vi "Insert LogData in Q.vi"(8 "error in (no error)":errorcluster, 10 "EventLog":T1) -> (0 "error out":errorcluster, 2 "# elements in queue":i32, 3 "EventLogDataQRef":refnum<queue>)   [LabVIEW 2022 SP3]
doc: "Developed by Kevin Thompson\nThompson Engineering, LLC\nkevin@thompsonengineering.net"
uses:
  TD EventLogData--cluster.ctl
  GBL DataQ Ref.vi
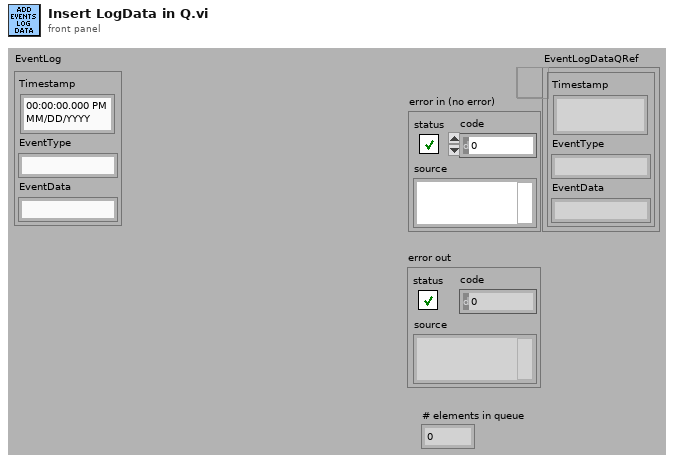
[diagram p1: front panel]
types:
  T1 = typedef "TD EventLogData--cluster.ctl" = cluster{"Timestamp":timestamp, "EventType":string, "EventData":string}
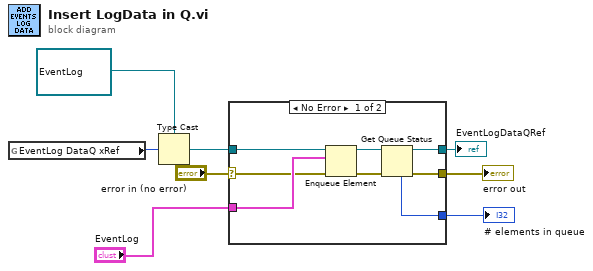
[diagram p0: block diagram]
diagram:
  n1 = global read "GBL DataQ Ref.vi" "EventLog DataQ xRef"() -> (w5:u32)
  n2 = Type Cast(type=refnum<queue> refnum ("EventLogDataQRef"), x=w5) -> (*(type *) &x=w6:refnum<queue>)
  n3 = case shown="No Error" "error in (no error)" {
    selector: "error in (no error)" -> [w13 w17]
    tunnel: w6 -> [w15 w18]
    tunnel: [w10 w17] -> w8
    tunnel: [w12 w18] -> w1
    tunnel: "EventLog" -> [w14 _]
    tunnel: [w9 _] -> w4
    frame No Error {
      n4 = Enqueue Element(queue=w15, element=w14, error in (no error)=w13) -> (queue out=w16:refnum<queue>, error out=w11:errorcluster)  [unwired: 1 in, 1 out]
      n5 = Get Queue Status(queue=w16, error in (no error)=w11) -> (queue out=w12:refnum<queue>, error out=w10:errorcluster, # elements in queue=w9:i32)  [unwired: 1 in, 5 out]
    }
    frame Error {
    }
  }
  "error out" <- w8
  "# elements in queue" <- w4
  "EventLogDataQRef" <- w1
